vi "UTIL_init_ini_resource_manager v1_0_0.vi"(8 "error in":errorcluster, 11 "Resource File":path) -> (0 "error out":errorcluster, 1 "Number of \nResources":i32, 2 "Resources":string[](array[string]))   [LabVIEW 2015]
doc: "This VI takes a file which contains all of the resources. The file must be tab deliminated with the first column being the resource name and the second being the resource value. The value can be a string or number, it can contain anything but tabs. All other columns are ignored. Comments can be stored in the third column.\n\nResource File: the path to the file which contians the resources.\n\nResource String: an array containing the entire line string excluding any comments.\n\nResources: an array contain only the name and value of each resource. The name is one array index lower than the associated value.\n\nNumber of Resources: the total number of resources.\n\nerror out: standard LabVIEW error cluster"
uses:
  <vilib>/Utility/config.llb/Read Key (String).vi
  <vilib>/Utility/config.llb/Read Key (Path).vi
  <vilib>/Utility/config.llb/NI_LVConfig.lvlib
panel:
  out "Percent Complete":dbl(slide) scale=0.0..100.0 scale format="%.1f"
  # "Initializing Resource Manager"
  # "Enter the name of the file containing the list of resource filenames"
  # "NOTE: Resource names\nare in index 0,2,4,6,..,etc\nand resource values are\nin index 1,3,5,7,..,etc!"
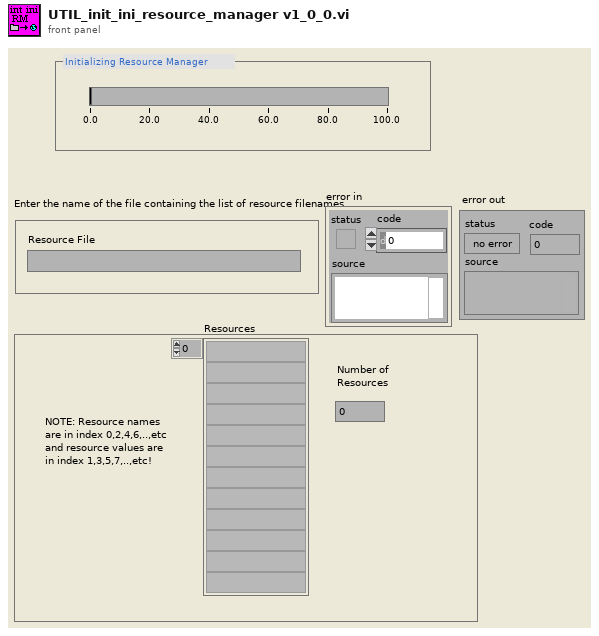
[diagram p1: front panel]
types:
  T1 = typedef "NI_LVConfig.lvlib/Config Data RefNum.ctl" = refnum<k1>
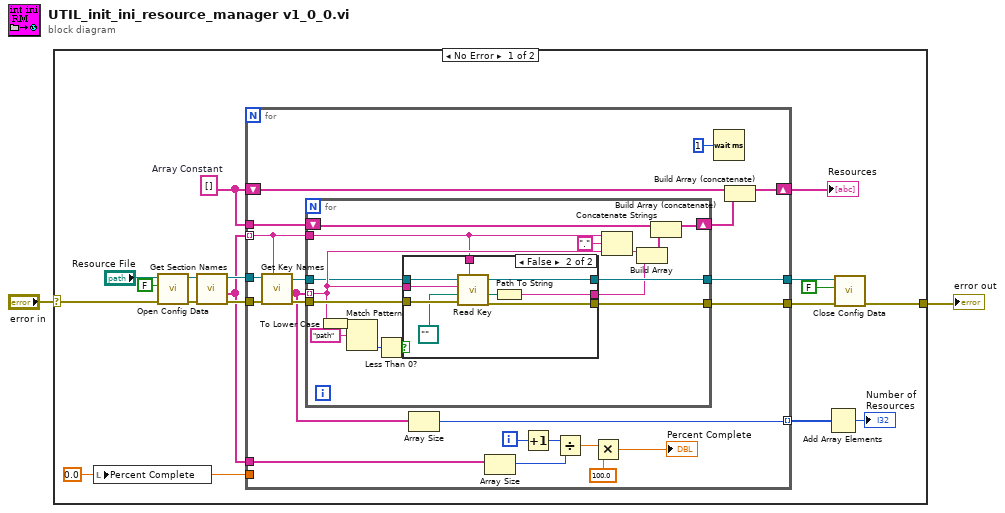
[diagram p0: block diagram]
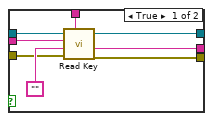
[diagram p2: hidden frame]
diagram:
  n1 = case shown="No Error" "error in" {
    selector: "error in" -> [w4 w74]
    tunnel: [w13 w74] -> w2
    frame No Error {
      w5 = 0.0 ("y")
      w10 = string[] []  # Array Constant
      n2 = local write "Percent Complete"(w5) -> ()
      n3 = call <vilib>:"Open Config Data.vi"("error in (no error)"=w4, "create file if necessary (T)"=FALSE, "configuration file path"="Resource File") -> ("error out"=w18:errorcluster, "refnum"=w19:T1)  [unwired: 6 in, 1 out]
      n4 = call <vilib>:"Get Section Names.vi"("error in (no error)"=w18, "refnum"=w19) -> ("error out"=w17:errorcluster, "section names"=w9:string[], "refnum out"=w16:T1)  [unwired: 7 out]
      n5 = for {
        tunnel: w17 -> [w40]
        tunnel: w16 -> [w39]
        tunnel: w9 -> [w38] mode=indexing
        tunnel: [w35] -> w15
        tunnel: [w34] -> w14
        shift-right: [w32] -> w12
        shift-left: w10 -> [w33]
        tunnel: w10 -> [w30]
        tunnel: w9 -> [w27]
        tunnel: [w28] -> w8 mode=indexing
        tunnel: w5 -> [_]
        i -> [w25]
        n6 = call <vilib>:"Get Key Names.vi"("section"=w38, "error in (no error)"=w40, "refnum"=w39) -> ("error out"=w36:errorcluster, "key names"=w29:string[], "refnum out"=w37:T1)  [unwired: 6 out]
        n7 = for {
          tunnel: w38 -> [w44]
          tunnel: w37 -> [w45]
          tunnel: w36 -> [w47]
          tunnel: w29 -> [w46] mode=indexing
          tunnel: [w42] -> w35
          tunnel: [w43] -> w34
          shift-right: [w53] -> w31
          shift-left: w30 -> [w52]
          n8 = To Lower Case(string=w46) -> (all lower case string=w50:string)
          n9 = Match Pattern(string=w50, regular expression="path") -> (offset past match=w49:i32)  [unwired: 4 out]
          n10 = Less Than 0?(x=w49) -> (x < 0?=w48:bool)
          n11 = case shown="False" w48 {
            tunnel: w47 -> [w61 w71]
            tunnel: w46 -> [w63 w73]
            tunnel: w45 -> [w62 w72]
            tunnel: w44 -> [w60 w70]
            tunnel: [w59 w69] -> w43
            tunnel: [w58 w68] -> w42
            tunnel: [w57 w65] -> w41
            frame True {
              n12 = call-poly <vilib>:"Read Key.vi"("section"=w60, "error in (no error)"=w61, "default value"="", "key"=w63, "refnum"=w62) -> ("error out"=w58:errorcluster, "value"=w57:string, "refnum out"=w59:T1)  [unwired: 1 in, 3 out]
            }
            frame False {
              n13 = call-poly <vilib>:"Read Key.vi"("section"=w70, "error in (no error)"=w71, "default value"=path "", "key"=w73, "refnum"=w72) -> ("error out"=w68:errorcluster, "value"=w67:path, "refnum out"=w69:T1)  [unwired: 4 out]
              n14 = Path To String(path=w67) -> (string=w65:string)
            }
          }
          n15 = Concatenate Strings(w44, "." ("Substring"), w46) -> (w55:string)
          n16 = Build Array(w55, w41) -> (w54:string[])
          n17 = Build Array (concatenate)(w52, w54) -> (w53:string[])
        }
        n18 = Array Size(array=w29) -> (size(s)=w28:i32)
        n19 = Array Size(array=w27) -> (size(s)=w26:i32)
        n20 = Increment(x=w25) -> (x+1=w21:i32)
        n21 = Divide(x=w21, y=w26) -> (x/y=w24:dbl)
        n22 = Multiply(x=w24, y=100.0) -> (x*y=→"Percent Complete":dbl)
        n23 = Wait (ms)(milliseconds to wait=u32 1) -> ()  [unwired: 1 out]
        n24 = Build Array (concatenate)(w33, w31) -> (w32:string[])
      }
      "Resources" <- w12
      n25 = Add Array Elements(numeric array=w8) -> (sum=→"Number of \nResources":i32)
      n26 = call <vilib>:"Close Config Data.vi"("error in (no error)"=w15, "write file if changed (T)"=FALSE ("write configuration file? (T)"), "refnum"=w14) -> ("error out"=w13:errorcluster)  [unwired: 8 out]
    }
    frame Error {
    }
  }
  "error out" <- w2
